vi "Get DDG External Output Enabled.vi"(10 "puiEnabled":u32, 11 "uiIndex":u32) -> (2 "puiEnabled out":u32, 3 "function return":u32)   [LabVIEW 2018, in "Copy of Andor SDK.lvlib"]
doc: "EXPNETTYPE unsigned int WINAPI GetDDGExternalOutputEnabled(at_u32 uiIndex, at_u32 * puiEnabled);"
uses:
  Copy of Andor SDK.lvlib
  <userlib>/Andor SDK/ATMCD32D.dll
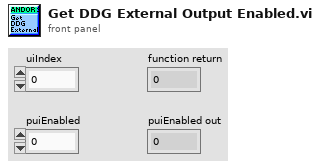
[diagram p1: front panel]
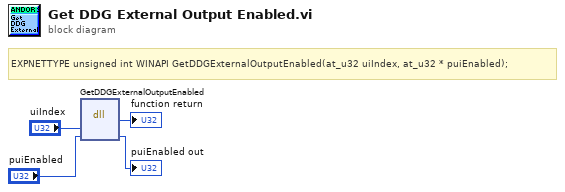
[diagram p0: block diagram]
diagram:
  # "EXPNETTYPE unsigned int WINAPI GetDDGExternalOutputEnabled(at_u32 uiIndex, at_u32 * puiEnabled);"
  n1 = dll-call lib="C:/Program Files (x86)/National Instruments/LabVIEW 2018/user.lib/Andor SDK/ATMCD32D.*" fn="GetDDGExternalOutputEnabled"("uiIndex"="uiIndex", "puiEnabled"="puiEnabled") -> (→"function return":u32, "puiEnabled"=→"puiEnabled out":u32)  [unwired: 4 in, 2 out]
